vi "Singleton Log Example.vi"() -> ()   [LabVIEW 2017, in "Logger Examples.lvlib"]
uses:
  Logger Examples.lvlib
  Source/Composed Log/Types/Log Level.ctl
  Source/Composed Log/LoggerReference/LoggerReference.lvclass/LoggerReference.ctl
  428adf5f-c5ee-4c09-9a5b-736284a89f6a.vi
  428adf5f-c5ee-4c09-9a5b-736284a89f6a.vi/f8c2809e-b149-4a86-9b79-c5596d2ebf16.vi
  Source/Composed Log/LoggerReference/Return Aggregate Queues.vi
  Source/Composed Log/LoggerReference/Add Aggregate Log.vi
  428adf5f-c5ee-4c09-9a5b-736284a89f6a.vi/f8c2809e-b149-4a86-9b79-c5596d2ebf16.vi/7431a603-47a1-4ce0-8b8b-a0fbd994e671.vi
  Source/Composed Log/LoggerReference/Log.vi
  Source/Composed Log/LoggerReference/Send Add Sink.vi
  Source/Composed Log/LoggerReference/Remove Stale Logs.vi
  Source/String Control Sink/String Control Sink.lvclass
  C:/CS/Internal/LabVIEW/Logger/Source/Composed Log/Log Sink/Log Sink.lvclass
  Source/Composed Log/Application Logger/Launch Worker Loop.vi
  Source/Composed Log/LoggerReference/Initialize Logger Instance.vi
  Source/Composed Log/Singleton Event Log/Logger Queue FGV.vi
  Source/Composed Log/IErrorFormat/IErrorFormat.lvclass
  Source/Composed Log/LoggerReference/LoggerReference.lvclass
  Source/Composed Log/Log Sink/Log Sink.lvclass
  Source/Composed Log/Singleton Event Log/Singleton Event Log.lvlib
  Source/Composed Log/Composed Log.lvlib
panel:
  in  "Event Level":T1(ring)
  out "Event Log":string
  in  "Data To Log":string
  in  "Source":string="User"
  in  "Log":bool
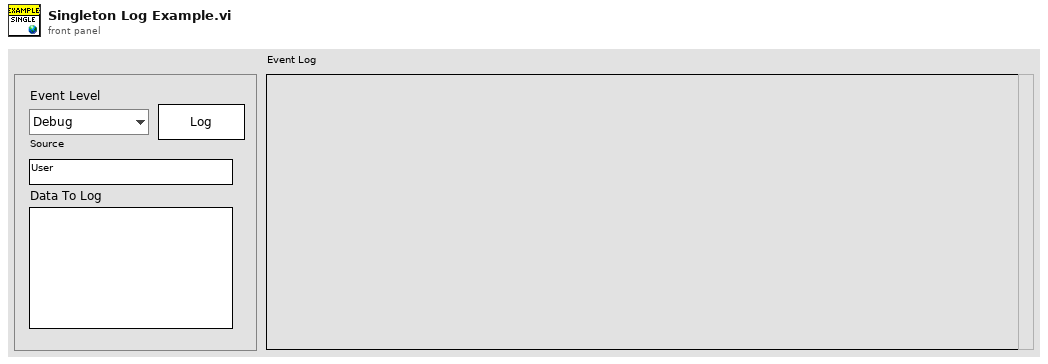
[diagram p1: front panel]
types:
  T1 = enum16{"Debug", "Info", "Warning", "Error", "Critical"}
  T2 = typedef "Composed Log.lvlib/Log Level.ctl" = enum16{"Debug", "Info", "Warning", "Error", "Critical"}
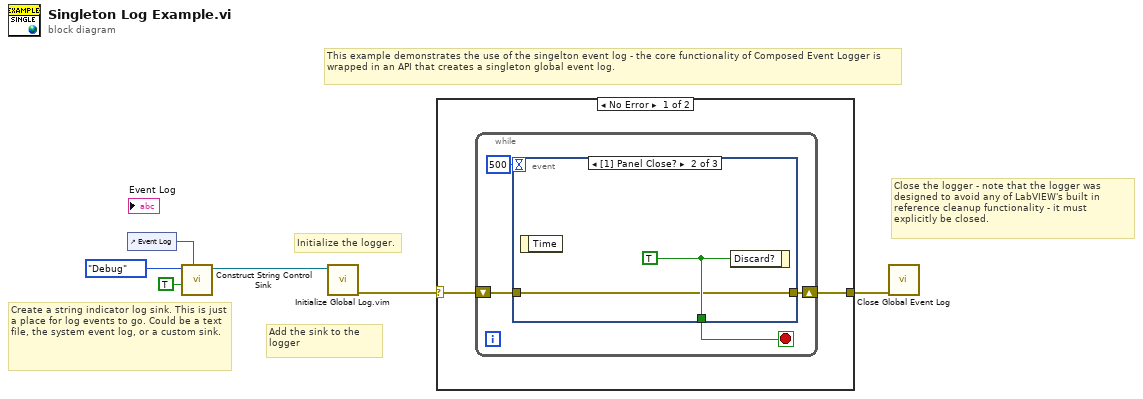
[diagram p0: block diagram]
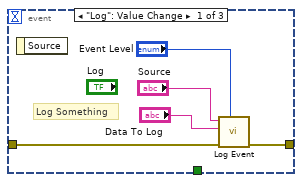
[diagram p2: hidden frame]
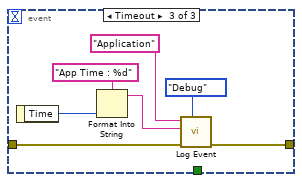
[diagram p3: hidden frame]
diagram:
  # "This example demonstrates the use of the singelton event log - the core functionality of Composed Event Logger is wrapped in an API that creates a singleton global event log."
  # "Add the sink to the logger"
  # "Close the logger - note that the logger was designed to avoid any of LabVIEW's built in reference cleanup functionality - it must explicitly be closed."
  # "Initialize the logger."
  # "Create a string indicator log sink. This is just a place for log events to go. Could be a text file, the system event log, or a custom sink."
  n1 = control-ref of="Event Log"() -> (w5:refnum<vi>)
  n2 = call "Construct String Control Sink.vi"("Str Refnum"=w5, "AutoScroll?(F)"=TRUE, "LogLevel"=Log_Level."Debug") -> ("String Control Sink out"=w6:refnum<class "String Control Sink.lvclass">)  [unwired: 8 in]
  n3 = call "Initialize Global Log.vim"("Log Sink(s)"=w6) -> ("error out"=w2:errorcluster)  [unwired: 9 in, 1 out]
  n4 = case shown="No Error" w2 {
    selector: w2 -> [w8 w27]
    tunnel: [w7 w27] -> w1
    frame No Error {
      n5 = while {
        shift-right: [w9] -> w7
        shift-left: w8 -> [w10]
        stop <- w12 stop-if-true
        n6 = event shown="[1] Panel Close?" {
          selector: _ -> [_ _ _]
          dyn-events: _ -> [_ _ _]
          timeout: 500 -> [_ _ _]
          tunnel: [_ w19 _] -> w12
          tunnel: w10 -> [w14 w18 w25]
          tunnel: [w13 w18 w24] -> w9
          event "Log": Value Change {
            # "Log Something"
            n7 = event-data() -> ()  [unwired: 1 in, 1 out]
            n8 = call "Log Event.vi"("Event Level"="Event Level", "error in (no error)"=w14, "Data To Log"="Data To Log", "SourceID"="Source") -> ("error out"=w13:errorcluster)  [unwired: 7 in]
          }
          event Panel Close? {
            w19 = TRUE ("Discard?")
            n9 = event-data() -> ()  [unwired: 1 in, 1 out]
            n10 = event-data("Discard?"=w19) -> ()  [unwired: 1 in, 1 out]
          }
          event Timeout {
            n11 = event-data() -> ("Time"=w22:u32)  [unwired: 1 in]
            n12 = Format Into String(format string="App Time : %d", w22) -> (resulting string=w20:string)  [unwired: 2 in, 1 out]
            n13 = call "Log Event.vi"("Event Level"=Log_Level."Debug", "error in (no error)"=w25, "Data To Log"=w20, "SourceID"="Application") -> ("error out"=w24:errorcluster)  [unwired: 7 in]
          }
        }
      }
    }
    frame Error {
    }
  }
  n14 = call "Close Global Event Log.vi"("error in (no error)"=w1) -> ()  [unwired: 10 in, 1 out]
